vi "multiply_size_by.vi"(9 "mutiply":u64, 10 "in":T1[](array[typedef])) -> (2 "out":T1[](array[typedef]))   [LabVIEW 2023]
uses:
  data_type/pixel/pixel.ctl
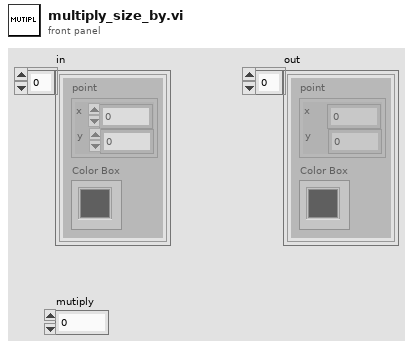
[diagram p1: front panel]
types:
  T1 = typedef "pixel.ctl" = cluster{"point":cluster{"x":i16, "y":i16}, "Color Box":u32}
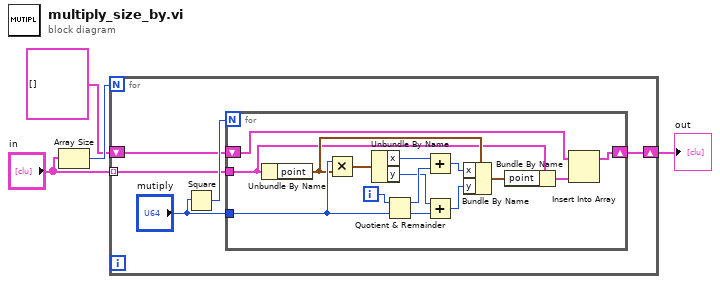
[diagram p0: block diagram]
diagram:
  n1 = Array Size(array="in") -> (size(s)=w4:i32)
  n2 = for {
    N: w4 -> [_]
    tunnel: "in" -> [w6] mode=indexing
    shift-right: [w7] -> w1
    shift-left: T1[] [] ("in") -> [w8]
    n3 = Square(x="mutiply") -> (x^2=w9:u64)
    n4 = for {
      N: w9 -> [_]
      shift-right: [w10] -> w7
      shift-left: w8 -> [w17]
      tunnel: w6 -> [w13]
      tunnel: "mutiply" -> [w22]
      i -> [w23]
      n5 = Unbundle By Name(w13) -> ("point"=w16:cluster{"x":i16, "y":i16})
      n6 = Multiply(x=w22, y=w16) -> (x*y=w24:cluster{"x":u64, "y":u64})
      n7 = Unbundle By Name(w24) -> ("x"=w20:u64, "y"=w19:u64)
      n8 = Quotient & Remainder(x=w23, y=w22) -> (x-y*floor(x/y)=w21:u64, floor(x/y)=w18:u64)
      n9 = Add(x=w20, y=w21) -> (x+y=w15:u64)
      n10 = Add(x=w19, y=w18) -> (x+y=w14:u64)
      n11 = Bundle By Name(cluster=w16, "x"=w15, "y"=w14) -> (w12:cluster{"x":i16, "y":i16})
      n12 = Bundle By Name(cluster=w13, "point"=w12) -> (w11:T1)
      n13 = Insert Into Array(array=w17, new element=w11) -> (w10:T1[])  [unwired: 1 in]
    }
  }
  "out" <- w1
